vi "Core Write DAQ FIFO.vi"(8 "error in (no error)":errorcluster, 10 "Data In":T1[](array[typedef]), 11 "CIFFIFO in":refnum<class "CIF_CIPC_Fifo_DAQ.lvclass">) -> (0 "error out":errorcluster, 2 "Data Out":T1[](array[typedef]), 3 "CIFFIFO out":refnum<class "CIF_CIPC_Fifo_DAQ.lvclass">)   [LabVIEW 2021, in "CIF_CIPC_Fifo_DAQ.lvclass"]
uses:
  CIF_CIPC_Fifo_DAQ.lvclass
  D:/dev/Packages/CIF_Channels_Core/src/CIFChannels/CIFChannels.lvclass
  D:/dev/Packages/CIF_Channels_Core/src/CIPC_Channels/CIF_CIPC_Chan/CIF_CIPC_Chn.lvclass
  CIFChannels/CIFChannels.lvclass/CIFChannels.ctl
  CIF_CIPC_Chan/CIF_CIPC_Chn.lvclass/CIF_CIPC_Chn.ctl
  <vilib>/CIF Foundation/CIF Utilities/Statistics/I64/Stats_I64_CIF_U.lvclass/Stats_I64_CIF_U.ctl
  1bad10da-a98b-49ee-b03a-18b497e396df.vi
  70f860b1-5d4a-43dc-b0c2-c9446e8447f7.vi
  CIFChannels/Accessors/Read FIFO Header.vi
  <vilib>/CIF Foundation/CIF Utilities/Statistics/I64/X1 minus X0.vi
  <vilib>/CIF Foundation/CIF Utilities/Time/System Time/Get System Time.vi
  <vilib>/CIF Foundation/CIF CIPC/SubVIs/Check Error.vi
  <vilib>/CIF Foundation/CIF CIPC/SubVIs/Notify Of New Write.vi
  <vilib>/CIF Foundation/CIF CIPC/SubVIs/Get dll Path.vi
  <vilib>/CIF Foundation/CIF CIPC/SubVIs/Get Element Write Position.vi
  <vilib>/CIF Foundation/CIF Utilities/Statistics/I64/X1 minus X0.vi/dfabcf33-0dbc-4041-80a5-3dc0c86d2989.vi
  <vilib>/CIF Foundation/CIF Utilities/Time/System Time/LabVIEW Time to TAI Time.vi
  <vilib>/CIF Foundation/CIF Utilities/Statistics/I64/X1 minus X0.vi/dfabcf33-0dbc-4041-80a5-3dc0c86d2989.vi/9eb60a9a-770f-4d2d-8b3f-8465c267ecc9.vi
  <vilib>/Utility/error.llb/Trim Whitespace.vi
  <vilib>/Utility/error.llb/Error Cluster From Error Code.vi
  CIF_CIPC_Fifo_DAQ.lvclass/CIF_CIPC_Fifo_DAQ.ctl
  CIFChannels/CIFChannels.lvclass
  CIF_CIPC_Chan/CIF_CIPC_Chn.lvclass
  D:/dev/Packages/CIF_Channels_Core/src/CIPC_Channels/FIFO_DAQ/CIF_CIPC_Fifo_DAQ.lvclass
  ChannelCommon/typedef/Datatype Waveform.ctl
  ChannelCommon/ChannelCommon.lvlib
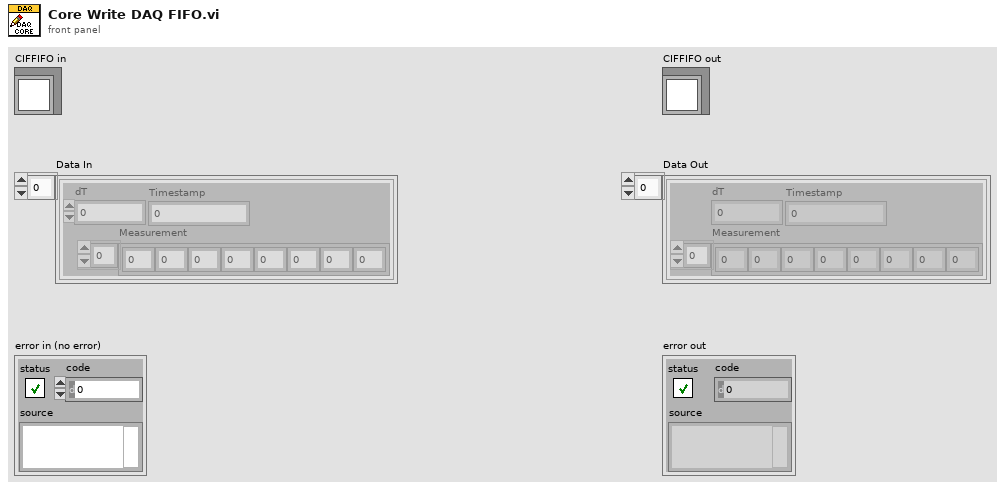
[diagram p1: front panel]
types:
  T1 = typedef "ChannelCommon.lvlib/Datatype Waveform.ctl" = cluster{"Measurement":dbl[], "dT":dbl, "Timestamp":i64}
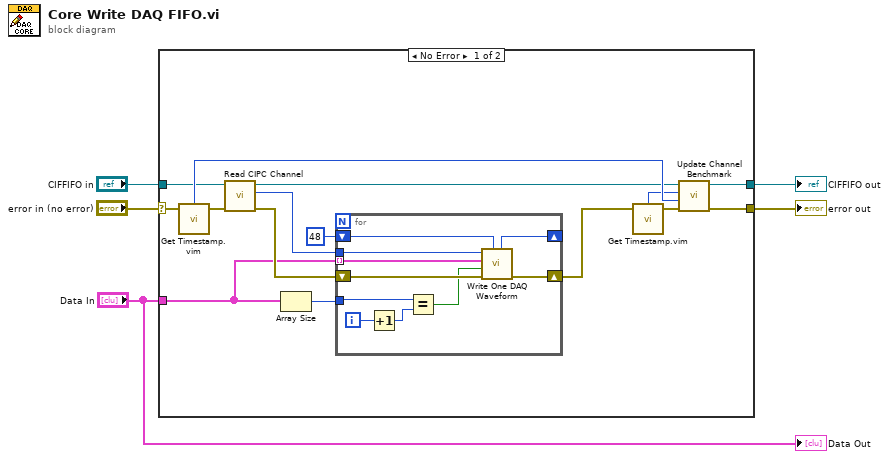
[diagram p0: block diagram]
diagram:
  n1 = case shown="No Error" "error in (no error)" {
    selector: "error in (no error)" -> [w16 w32]
    tunnel: [w20 w32] -> w4
    tunnel: [w19 w31] -> w2
    tunnel: "CIFFIFO in" -> [w10 w31]
    tunnel: "Data In" -> [w7 _]
    frame No Error {
      n2 = call "Get Timestamp.vim"("Anything in"=w16) -> ("Time (ns)"=w18:i64, "Anything out"=w9:errorcluster)  [unwired: 2 in]
      n3 = call "Read CIPC Channel.vi"("error in (no error)"=w9, "CIFTag in"=w10) -> ("error out"=w12:errorcluster, "CIPC Channel"=w13:u64, "CIFTag out"=w14:refnum<class "CIF_CIPC_Fifo_DAQ.lvclass">)  [unwired: 7 in]
      n4 = Array Size(array=w7) -> (size(s)=w6:i32)
      n5 = for {
        tunnel: w13 -> [w30]
        tunnel: w7 -> [w24] mode=indexing
        shift-right: [w29] -> w11
        shift-left: w12 -> [w25]
        shift-right: [w22] -> _
        shift-left: u32 48 ("y") -> [w23]
        tunnel: w6 -> [w27]
        i -> [w28]
        n6 = Increment(x=w28) -> (x+1=w26:i32)
        n7 = Equal?(x=w27, y=w26) -> (x = y?=w21:bool)
        n8 = call "Write One DAQ Waveform.vi"("Offset in"=w23, "error in (no error)"=w25, "Last Waveform"=w21, "Waveform Datatype"=w24, "CIPC Channel"=w30) -> ("error out"=w29:errorcluster, "Offset out"=w22:u32)  [unwired: 5 in]
      }
      n9 = call "Get Timestamp.vim"("Anything in"=w11) -> ("Time (ns)"=w17:i64, "Anything out"=w15:errorcluster)  [unwired: 2 in]
      n10 = call "Update Channel Benchmark.vi"("error in (no error)"=w15, "X0"=w18, "X1"=w17, "CIFChannels in"=w14) -> ("error out"=w20:errorcluster, "CIFChannels out"=w19:refnum<class "CIF_CIPC_Fifo_DAQ.lvclass">)  [unwired: 6 in]
    }
    frame Error {
    }
  }
  "error out" <- w4
  "CIFFIFO out" <- w2
  "Data Out" <- "Data In"
